vi "BuildCustomDashBoardData.vi"() -> ()   [LabVIEW 2013]
doc: "This VI builds data and sends it back to the dashboard PC program. By default it sends back the raw values for the first analog, digital, and solenoid module. Modify it to send back the data you want to view. Consider adding higher level data to the Dashboard Datatype.ctl and to this VI. Then update the Dashboard to display the data however you like.\n\nThis software is licensed. Open the labview\\readme\\WPI Robotics Library Open Source License.txt file for more information."
uses:
  typedefs/Dashboard/DashboardEnable.ctl
  <vilib>/Rock Robotics/SystemInterfaces/Typedef/FPGA_TypedefDigitalModule.ctl
  <vilib>/Rock Robotics/WPI/DriverStation/WPI_DriverStationDigitalData.ctl
  typedefs/fg_typedef.ctl
  typedefs/Dashboard/misc dash data.ctl
  typedefs/Dashboard/dashboard safety status data.ctl
  typedefs/Dashboard/drive safety.ctl
  typedefs/Dashboard/dash error type def.ctl
  <vilib>/Rock Robotics/SystemInterfaces/System/FPGA_SystemGet.vi
  <vilib>/Rock Robotics/WPI/Compressor/WPI_CompressorGetSetRefNum.vi
  <vilib>/NI_Real-Time Target Support.lvlib
  typedefs/State Machine/subStates.ctl
  typedefs/Dashboard/custom dash data.ctl
  typedefs/Dashboard/Dashboard Datatype.ctl
panel:
  out "Errors":errorcluster
  # "Generate Dashboard Data and Send it"
  # "Note: Test code calls some dashboard data, which is gotten there not here"
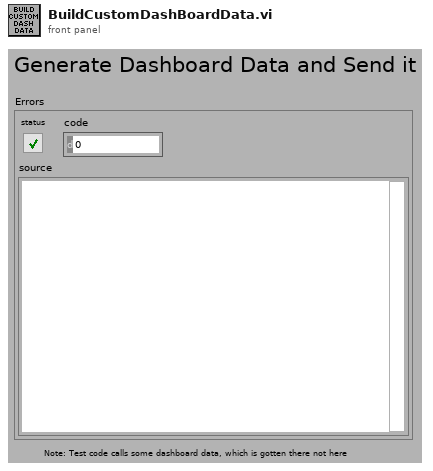
[diagram p1: front panel]
types:
  T1 = typedef "Dashboard Datatype.ctl" = cluster{cluster{"AnalogModule[0]":cluster{"Channel[0]":sgl, "Channel[1]":sgl, "Channel[2]":sgl, "Channel[3]":sgl, "Channel[4]":sgl, "Channel[5]":sgl, "Channel[6]":sgl, "Channel[7]":sgl}, "AnalogModule[1]":cluster{"Channel[0]":sgl, "Channel[1]":sgl, "Channel[2]":sgl, "Channel[3]":sgl, "Channel[4]":sgl, "Channel[5]":sgl, "Channel[6]":sgl, "Channel[7]":sgl}}, cluster{"DigitalModule[0]":T2, "DigitalModule[1]":T2}, "Solenoid":u8}
  T2 = typedef "WPI_DriverStationDigitalData.ctl" = cluster{"Relay Fwd":u8, "Relay Rev":u8, "GPIO":u16, "GPIO_OE":u16, "PWM":cluster{"PWM[0]":u8, "PWM[1]":u8, "PWM[2]":u8, "PWM[3]":u8, "PWM[4]":u8, "PWM[5]":u8, "PWM[6]":u8, "PWM[7]":u8, "PWM[8]":u8, "PWM[9]":u8}}
  T3 = typedef "custom dash data.ctl" = cluster{"Motors":cluster{"Pickup Motor":dbl, "Pickup Belt":dbl, "Pickup Distance ":dbl, "Pickup Rate":dbl, "Right Motor Rate":dbl, "Left Motor Rate":dbl, "Right Motor Distance":dbl, "Left Motor Distance":dbl}, "substates":cluster{"Latch":T4, "Pickup Arm":T4, "Belts":T4, "Shooter":T4, "Drive":T4}, "Safeties":cluster{"Arm Safety":bool, "Arm Limit":bool}, "Performance":cluster{"CPU Usage":dbl, "Vision mSPI":u32, "Main mSPI":u32}, "Vision Enabled?":bool, "Can Shoot Safely?":bool, "Timeout Error":cluster{"# of Timeouts":u32, "Time Out Error This Match":bool}, "Error FG Data":cluster{"Errors Present":bool, "Errors":string}, "Vision Data":cluster{"Hot Goal Present?":bool, "distance":dbl}}
  T4 = typedef "subStates.ctl" = enum16{"null", "wait", "driver control", "auto", "manual override", "hold position", "rotate", "pickup", "pass", "recover pass", "load", "goto shoot", "shoot high goal", "shoot low goal", "cancel arm", "cancel shooter", "end", "test"}
  T5 = typedef "fg_typedef.ctl" = enum16{"Get", "Set"}
  T6 = cluster{"# of Timeouts":u32, "Time Out Error This Match":bool}
  T7 = typedef "FPGA_TypedefDigitalModule.ctl" = enum16{"Digital Module 1", "Digital Module 2"}
  T8 = typedef "misc dash data.ctl" = cluster{"Total (%)":dbl, "Vision mSPI":u32, "Main mSPI":u32, "Vision":cluster{"Hot Goal Present?":bool, "distance":dbl}, "Enabled?":bool, "Arm Safety Data":T9, "Drive Safety Data":T10, "TeleOp Elapsed Seconds":dbl}
  T9 = typedef "dashboard safety status data.ctl" = cluster{"At Distance Limit":bool, "No Rate Read":bool, "Encoder Failure":bool, "Encoder Directional Issue":bool}
  T10 = typedef "drive safety.ctl" = cluster{"Left - Encoder Failure":bool, "Left - No Rate Read":bool, "Right - Encoder Failure":bool, "Right - No Rate Read":bool}
  T11 = typedef "dash error type def.ctl" = cluster{"Timeout Data":cluster{"# of Timeouts":u32, "Time Out Error This Match":bool}, "Can Shoot Safely?":bool}
  T12 = typedef "DashboardEnable.ctl" = cluster{"Analog Module 1":bool[], "Analog Module 2":bool[], "Digital Module 1":bool, "Digital Module 2":bool, "Solenoid Module":bool}
  T13 = cluster{"AnalogModule[0]":cluster{"Channel[0]":sgl, "Channel[1]":sgl, "Channel[2]":sgl, "Channel[3]":sgl, "Channel[4]":sgl, "Channel[5]":sgl, "Channel[6]":sgl, "Channel[7]":sgl}, "AnalogModule[1]":cluster{"Channel[0]":sgl, "Channel[1]":sgl, "Channel[2]":sgl, "Channel[3]":sgl, "Channel[4]":sgl, "Channel[5]":sgl, "Channel[6]":sgl, "Channel[7]":sgl}}
  T14 = cluster{"DigitalModule[0]":T2, "DigitalModule[1]":T2}
  T15 = typedef "vision data.ctl" = cluster{"x":dbl, "y":dbl, "area":dbl, "width":dbl, "height":dbl, "Hot Goal Present?":bool, "distance":dbl}
  T16 = cluster{"Channel[0]":sgl, "Channel[1]":sgl, "Channel[2]":sgl, "Channel[3]":sgl, "Channel[4]":sgl, "Channel[5]":sgl, "Channel[6]":sgl, "Channel[7]":sgl}[]
  T17 = cluster{"Channel[0]":sgl, "Channel[1]":sgl, "Channel[2]":sgl, "Channel[3]":sgl, "Channel[4]":sgl, "Channel[5]":sgl, "Channel[6]":sgl, "Channel[7]":sgl}
  T18 = cluster{"AnalogModule[0][0]":sgl, "AnalogModule[0][1]":sgl, "AnalogModule[0][2]":sgl, "AnalogModule[0][3]":sgl, "AnalogModule[0][4]":sgl, "AnalogModule[0][5]":sgl, "AnalogModule[0][6]":sgl, "AnalogModule[0][7]":sgl}
  T19 = cluster{"[0]":cluster{"Channel[0]":sgl, "Channel[1]":sgl, "Channel[2]":sgl, "Channel[3]":sgl, "Channel[4]":sgl, "Channel[5]":sgl, "Channel[6]":sgl, "Channel[7]":sgl}, "[1]":cluster{"Channel[0]":sgl, "Channel[1]":sgl, "Channel[2]":sgl, "Channel[3]":sgl, "Channel[4]":sgl, "Channel[5]":sgl, "Channel[6]":sgl, "Channel[7]":sgl}}
  T20 = typedef "FPGA_DIODevRef.ctl" = cluster{"DevStatus":errorcluster, "Module":T7}
  T21 = cluster{"[0]":u8, "[1]":u8, "[2]":u8, "[3]":u8, "[4]":u8, "[5]":u8, "[6]":u8, "[7]":u8, "[8]":u8, "[9]":u8}
  T22 = typedef "FPGA_SolenoidDevRef.ctl" = cluster{"DevStatus":errorcluster, "Module":T23}
  T23 = typedef "FPGA_TypedefSolenoidModule.ctl" = enum16{"Solenoid Module 1", "Solenoid Module 2"}
  T24 = cluster{"Pickup Motor":dbl, "Pickup Belt":dbl, "Pickup Distance ":dbl, "Pickup Rate":dbl, "Right Motor Rate":dbl, "Left Motor Rate":dbl, "Right Motor Distance":dbl, "Left Motor Distance":dbl}
  T25 = cluster{"CPU Usage":dbl, "Vision mSPI":u32, "Main mSPI":u32}
  T26 = cluster{"Hot Goal Present?":bool, "distance":dbl}
  T27 = typedef "WPI_EncoderDevRef.ctl" = cluster{"DevStatus":errorcluster, "EncoderIndex":T28, "CounterIndex":T29, "DistancePerCount":dbl, "Decoding Type":T30}
  T28 = typedef "FPGA_EncoderIdx.ctl" = enum8{"Enc 0", "Enc 1", "Enc 2", "Enc 3", "Invalid"}
  T29 = typedef "FPGA_CounterCtrSystemIndex.ctl" = enum8{"Ctr 0", "Ctr 1", "Ctr 2", "Ctr 3", "Ctr 4", "Ctr 5", "Ctr 6", "Ctr 7", "Invalid"}
  T30 = typedef "WPI_EncoderType.ctl" = enum16{"1x", "2x", "4x"}
  T31 = typedef "WPI_MotorControlDeviceRef.ctl" = cluster{"DeviceStatus":errorcluster, "Type":enum16{"PWM", "CAN"}, "PWM":cluster{"Digital Module":T7, "PWM Channel":T32, "DeadBand":T33}, "CAN":cluster{"Device Number":u8, "Control Mode":T34, "Semaphore":T35, "Max Vout":dbl}, "Invert":bool, "TransformRef":T36, "InvTransformRef":T36}
  T32 = typedef "FPGA_DIOPWMChannel.ctl" = enum8{"PWM 1", "PWM 2", "PWM 3", "PWM 4", "PWM 5", "PWM 6", "PWM 7", "PWM 8", "PWM 9", "PWM 10", "Invalid"}
  T33 = typedef "WPI_PWMDeadband.ctl" = cluster{"Name":string, "maxPositivePwm":i32, "minPositivePwm":i32, "centerPwm":i32, "maxNegativePwm":i32, "minNegativePwm":i32, "angularRange":u16}
  T34 = typedef "WPI_CANJaguar_ControlMode.ctl" = enum8{"Percent VBus", "Current", "Speed", "Position", "Voltage"}
  T35 = typedef "Semaphore RefNum" = refnum<k1>
  T36 = typedef "WPI_PWMTransform_ConPane.ctl" = refnum<vi>
  T37 = typedef "NI_Real-Time Target Support.lvlib/RT CPU Load.ctl" = cluster{"Total (%)":dbl, "Time Critical (%)":dbl, "Timed Structures (%)":dbl, "High (%)":dbl, "Above Normal (%)":dbl, "Normal (%)":dbl, "Background (%)":dbl, "Idle (%)":dbl, "ISR (%)":dbl}
  T38 = cluster{"Vision mSPI":u32, "Main mSPI":u32, "Dash mSPI":u32}
  T39 = typedef "WPI_CompressorDevRef.ctl" = cluster{"DevStatus":errorcluster, "DigitalInputDevRef":T40, "RelayDevRef":T42}
  T40 = typedef "WPI_DigitalInputDevRef.ctl" = cluster{"DevStatus":errorcluster, "DIO Channel":T41, "Digital Module":T7}
  T41 = typedef "FPGA_DIOChannel.ctl" = enum8{"DIO 1", "DIO 2", "DIO 3", "DIO 4", "DIO 5", "DIO 6", "DIO 7", "DIO 8", "DIO 9", "DIO 10", "DIO 11", "DIO 12", "DIO 13", "DIO 14", "Invalid"}
  T42 = typedef "WPI_RelayDevRef.ctl" = cluster{"DevStatus":errorcluster, "Relay Channel":T43, "Digital Module":T7, "Relay Direction":T44}
  T43 = typedef "FPGA_DIORelayChannel.ctl" = enum8{"Relay 1", "Relay 2", "Relay 3", "Relay 4", "Relay 5", "Relay 6", "Relay 7", "Relay 8", "Invalid"}
  T44 = typedef "WPI_RelayDirection.ctl" = enum16{"Both directions", "Forward only", "Reverse only"}
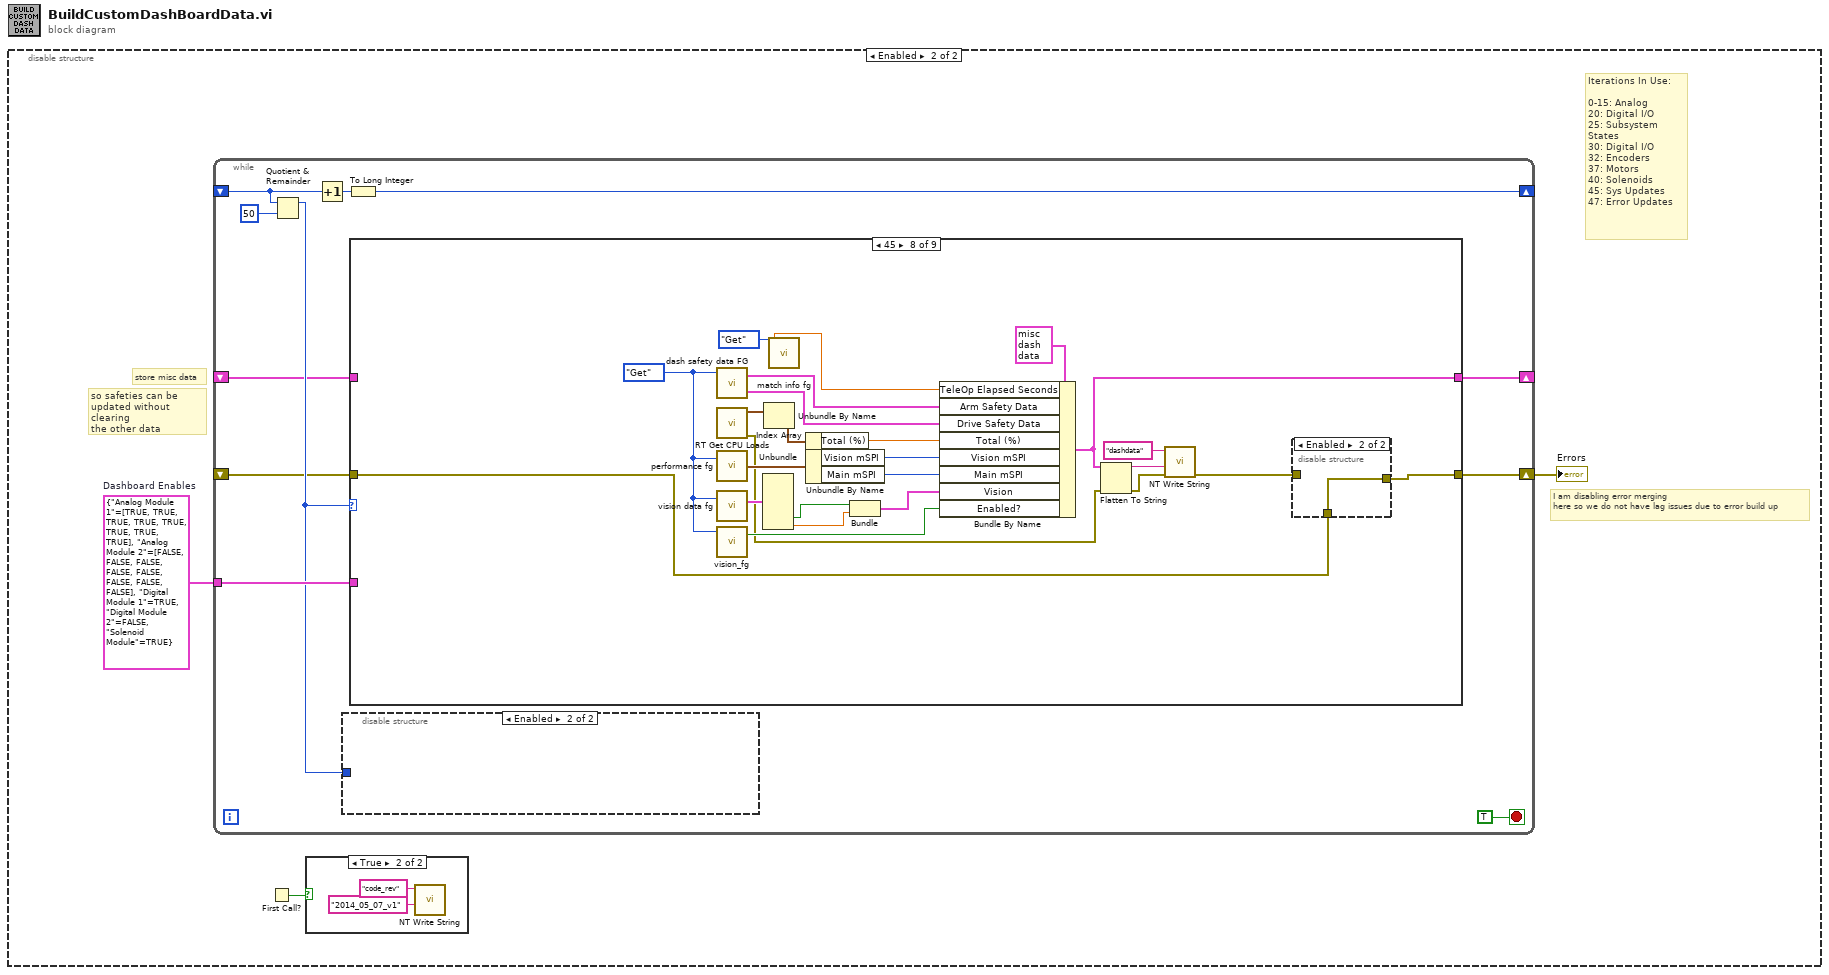
[diagram p0: block diagram]
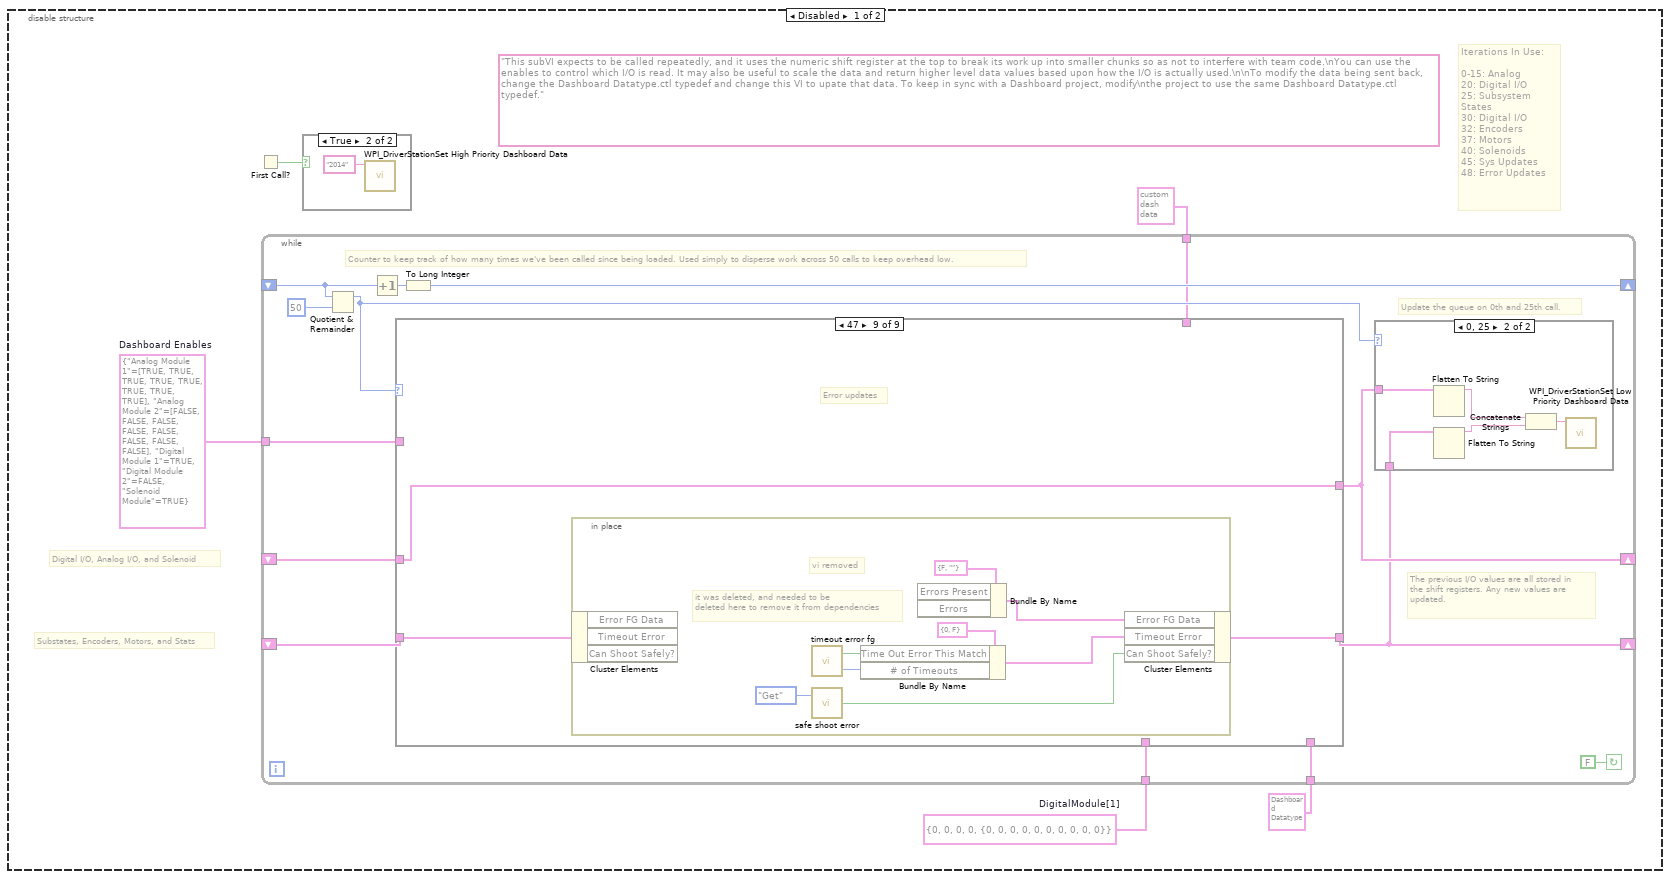
[diagram p2: hidden frame]
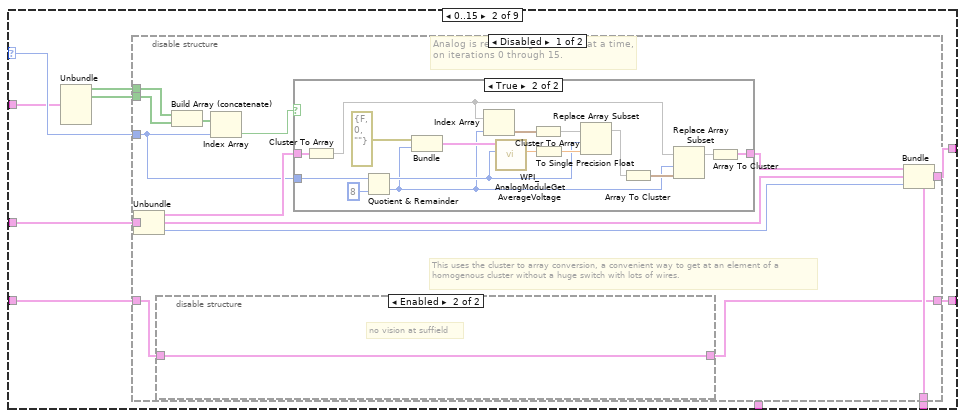
[diagram p6: hidden frame]
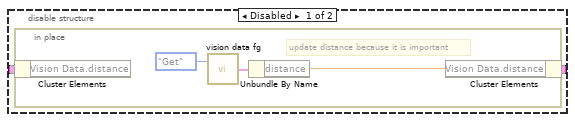
[diagram p8: hidden frame]
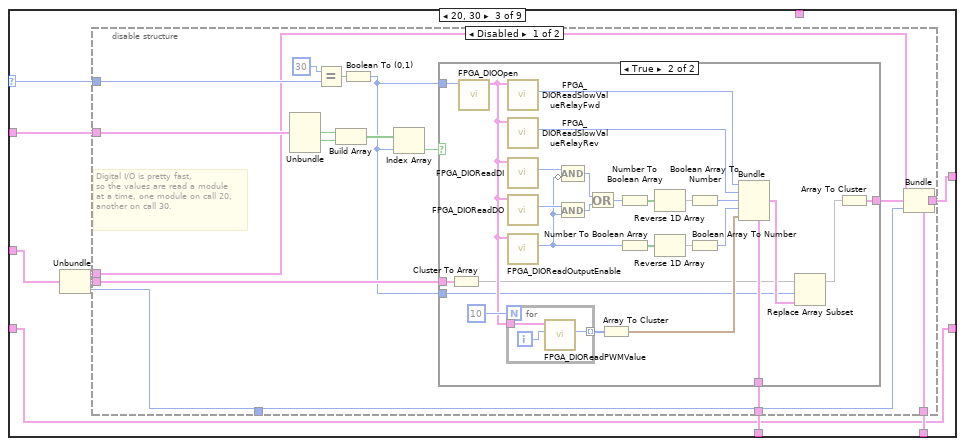
[diagram p10: hidden frame]
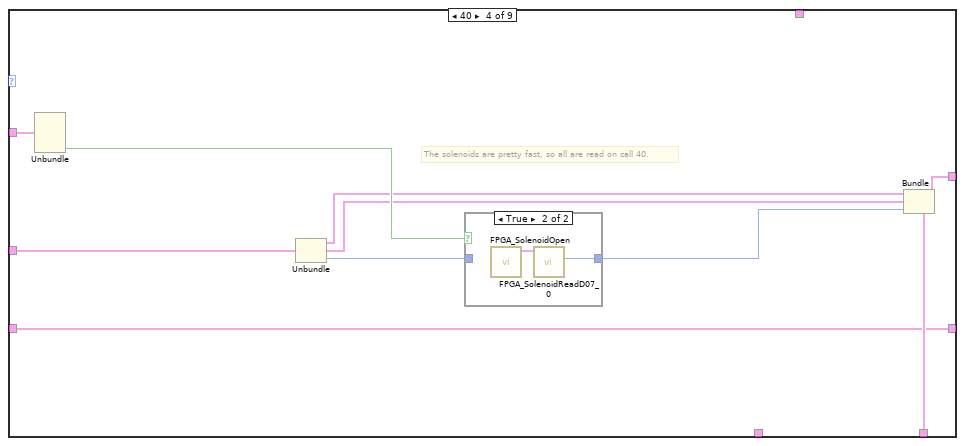
[diagram p13: hidden frame]
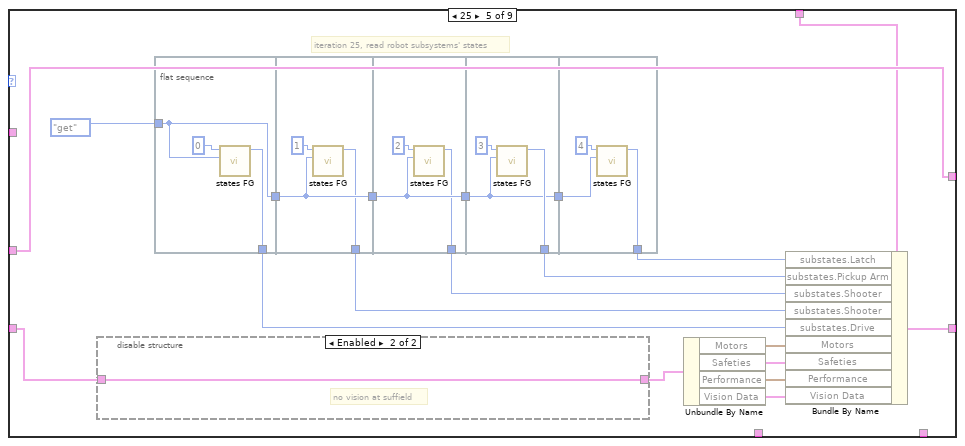
[diagram p15: hidden frame]
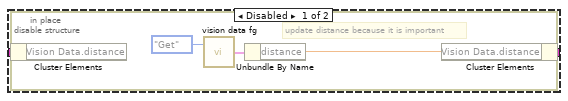
[diagram p16: hidden frame]
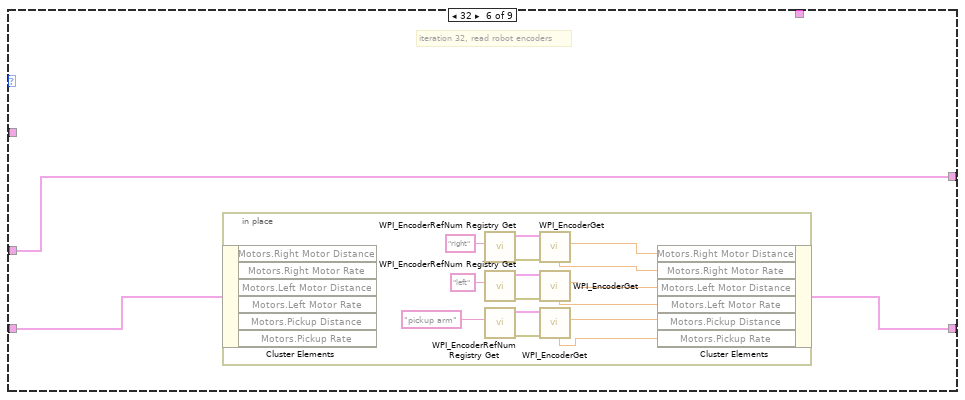
[diagram p17: hidden frame]
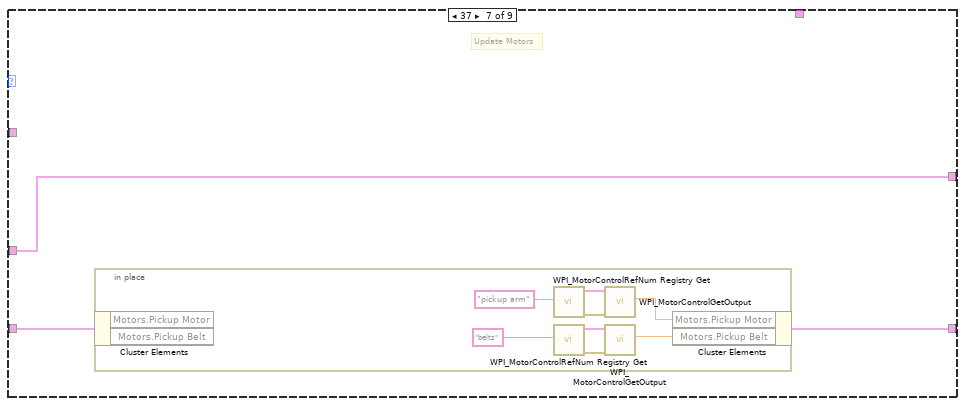
[diagram p18: hidden frame]
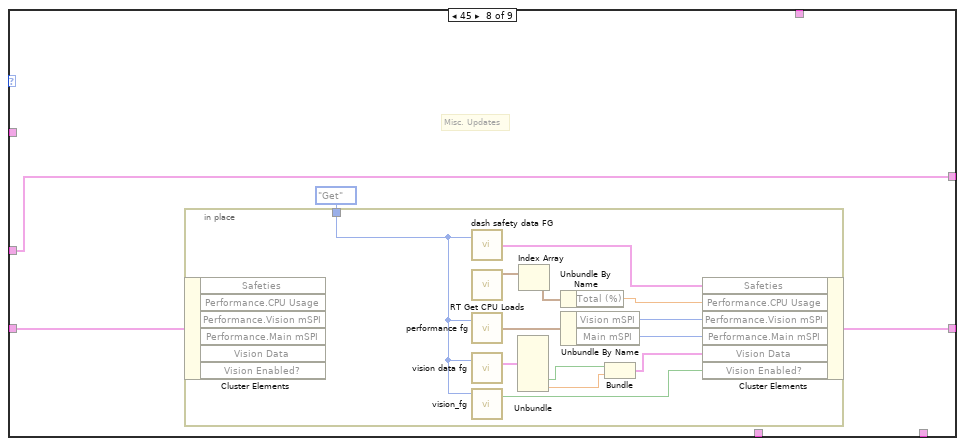
[diagram p19: hidden frame]
diagram:
  n1 = disable-structure shown="Enabled" {
    frame Disabled {
      w1 = T12 {"Analog Module 1"=[TRUE, TRUE, TRUE, TRUE, TRUE, TRUE, TRUE, TRUE], "Analog Module 2"=[FALSE, FALSE, FALSE, FALSE, FALSE, FALSE, FALSE, FALSE], "Digital Module 1"=TRUE, "Digital Module 2"=FALSE, "Solenoid Module"=TRUE}  # Dashboard Enables
      w2 = T2 {"Relay Fwd"=0, "Relay Rev"=0, "GPIO"=0, "GPIO_OE"=0, "PWM"={"PWM[0]"=0, "PWM[1]"=0, "PWM[2]"=0, "PWM[3]"=0, "PWM[4]"=0, "PWM[5]"=0, "PWM[6]"=0, "PWM[7]"=0, "PWM[8]"=0, "PWM[9]"=0}}  # DigitalModule[1]
      (unwired) "This subVI expects to be called repeatedly, and it uses the numeric shift register at the top to break its work up into smaller chunks so as not to interfere with team code.\nYou can use the enables to control which I/O is read. It may also be useful to scale the data and return higher level data values based upon how the I/O is actually used.\n\nTo modify the data being sent back, change the Dashboard Datatype.ctl typedef and change this VI to upate that data. To keep in sync with a Dashboard project, modify\nthe project to use the same Dashboard Datatype.ctl typedef."
      # "Iterations In Use:\n\n0-15: Analog\n20: Digital I/O \n25: Subsystem States\n30: Digital I/O\n32: Encoders\n37: Motors\n40: Solenoids\n45: Sys Updates\n48: Error Updates"
      # "Substates, Encoders, Motors, and Stats"
      # "Digital I/O, Analog I/O, and Solenoid"
      n2 = First Call?() -> (First Call?: T/F=w3:bool)
      n3 = while {
        shift-right: [w13] -> _
        shift-left: _ -> [w15]
        shift-right: [w10] -> _
        shift-left: _ -> [w18]
        tunnel: w2 -> [w17]
        tunnel: T1 {{"AnalogModule[0]"={"Channel[0]"=0.0, "Channel[1]"=0.0, "Channel[2]"=0.0, "Channel[3]"=0.0, "Channel[4]"=0.0, "Channel[5]"=0.0, "Channel[6]"=0.0, "Channel[7]"=0.0}, "AnalogModule[1]"={"Channel[0]"=0.0, "Channel[1]"=0.0, "Channel[2]"=0.0, "Channel[3]"=0.0, "Channel[4]"=0.0, "Channel[5]"=0.0, "Channel[6]"=0.0, "Channel[7]"=0.0}}, {"DigitalModule[0]"={"Relay Fwd"=0, "Relay Rev"=0, "GPIO"=0, "GPIO_OE"=0, "PWM"={"PWM[0]"=0, "PWM[1]"=0, "PWM[2]"=0, "PWM[3]"=0, "PWM[4]"=0, "PWM[5]"=0, "PWM[6]"=0, "PWM[7]"=0, "PWM[8]"=0, "PWM[9]"=0}}, "DigitalModule[1]"={"Relay Fwd"=0, "Relay Rev"=0, "GPIO"=0, "GPIO_OE"=0, "PWM"={"PWM[0]"=0, "PWM[1]"=0, "PWM[2]"=0, "PWM[3]"=0, "PWM[4]"=0, "PWM[5]"=0, "PWM[6]"=0, "PWM[7]"=0, "PWM[8]"=0, "PWM[9]"=0}}}, "Solenoid"=0} ("Dashboard Data") -> [w12]
        tunnel: w1 -> [w11]
        shift-right: [w7] -> _
        shift-left: _ -> [w8]
        tunnel: T3 {"Motors"={"Pickup Motor"=0.0, "Pickup Belt"=0.0, "Pickup Distance "=0.0, "Pickup Rate"=0.0, "Right Motor Rate"=0.0, "Left Motor Rate"=0.0, "Right Motor Distance"=0.0, "Left Motor Distance"=0.0}, "substates"={"Latch"=enum."null", "Pickup Arm"=enum."null", "Belts"=enum."null", "Shooter"=enum."null", "Drive"=enum."null"}, "Safeties"={"Arm Safety"=FALSE, "Arm Limit"=FALSE}, "Performance"={"CPU Usage"=0.0, "Vision mSPI"=0, "Main mSPI"=0}, "Vision Enabled?"=FALSE, "Can Shoot Safely?"=FALSE, "Timeout Error"={"# of Timeouts"=0, "Time Out Error This Match"=FALSE}, "Error FG Data"={"Errors Present"=FALSE, "Errors"=""}, "Vision Data"={"Hot Goal Present?"=FALSE, "distance"=0.0}} ("Custom Dash Data") -> [w9]
        stop <- FALSE continue-if-true
        # "Counter to keep track of how many times we've been called since being loaded. Used simply to disperse work across 50 calls to keep overhead low."
        # "Update the queue on 0th and 25th call."
        # "The previous I/O values are all stored in\nthe shift registers. Any new values are\nupdated."
        n4 = Quotient & Remainder(x=w15, y=50) -> (x-y*floor(x/y)=w14:i32)  [unwired: 1 out]
        n5 = Increment(x=w15) -> (x+1=w20:i32)
        n6 = case shown="47" w14 {
          selector: w14 -> [_ w35 w82 _ _ _ _ _ _]
          tunnel: [w27 w31 w77 w136 w151 w184 w203 w214 w230] -> w10
          tunnel: w18 -> [w27 w30 w79 w138 w151 w184 w203 w214 w230]
          tunnel: w17 -> [_ _ w83 _ _ _ _ _ _]
          tunnel: w12 -> [_ w36 w78 w135 _ _ _ _ _]
          tunnel: w11 -> [_ w34 w81 w139 _ _ _ _ _]
          tunnel: w9 -> [_ _ _ _ w149 _ _ _ _]
          tunnel: [w26 w28 w76 w132 w150 w185 w202 w215 w231] -> w7
          tunnel: w8 -> [w26 w29 w76 w132 w145 w183 w201 w213 w229]
          frame Default {
            # "Don't update any I/O"
          }
          frame 0..15 {
            n7 = Unbundle(w34) -> ("Analog Module 1"=w33:bool[], "Analog Module 2"=w32:bool[])  [unwired: 3 out]
            n8 = disable-structure shown="Disabled" {
              disable-tunnel: w36 -> [w47 _]
              disable-tunnel: w35 -> [w45 _]
              disable-tunnel: w33 -> [w44 _]
              disable-tunnel: w32 -> [w43 _]
              disable-tunnel: [w42 _] -> w31
              disable-tunnel: w30 -> [w41 _]
              disable-tunnel: w29 -> [w38 _]
              disable-tunnel: [w37 _] -> w28
              frame Disabled {
                # "This uses the cluster to array conversion, a convenient way to get at an element of a\nhomogenous cluster without a huge switch with lots of wires."
                # "Analog is read a single channel at a time,\non iterations 0 through 15."
                n9 = Unbundle(w41) -> (w46:T13, w40:T14, "Solenoid"=w39:u8)
                n10 = disable-structure shown="Enabled" {
                  disable-tunnel: w38 -> [w69 w73]
                  disable-tunnel: [w68 w73] -> w37
                  frame Disabled {
                    n11 = in-place {
                      # "update distance because it is important"
                      n12 = in-place-cluster #1(w69) -> ()  [unwired: 1 out]
                      n13 = call "vision data fg.vi"("Menu"=fg_typedef."Get") -> ("Output"=w71:T15)  [unwired: 1 in]
                      n14 = Unbundle By Name(w71) -> ("distance"=w70:dbl)
                      n15 = in-place-cluster #1("Vision Data.distance"=w70) -> (w68:T3)
                    }
                  }
                  frame Enabled {
                    # "no vision at suffield"
                  }
                }
                n16 = Build Array (concatenate)(w44, w43) -> (w49:bool[])
                n17 = Index Array(array=w49, index=w45) -> (element=w50:bool)
                n18 = case shown="True" w50 {
                  tunnel: w45 -> [_ w58]
                  tunnel: [w51 w55] -> w48
                  tunnel: w46 -> [w51 w54]
                  frame False {
                  }
                  frame True {
                    n19 = Cluster To Array(cluster=w54) -> (array=w53:T16)
                    n20 = Quotient & Remainder(x=w58, y=8) -> (x-y*floor(x/y)=w57:i32, floor(x/y)=w52:i32)
                    n21 = Bundle("DevStatus"=errorcluster {"status"=FALSE, "code"=0, "source"=""}, w52) -> (w66:cluster{"DevStatus":errorcluster, i32})  [unwired: 1 out]
                    n22 = Index Array(array=w53, index=w52) -> (element=w60:T17)
                    n23 = call <vilib>:"WPI_AnalogModuleGetAverageVoltage.vi"("Channel"=w57, "AnalogModuleDevStatus"=w66) -> ("Average Voltage"=w63:dbl)  [unwired: 1 in, 8 out]
                    n24 = Cluster To Array(cluster=w60) -> (array=w59:sgl[])
                    n25 = To Single Precision Float(number=w63) -> (single precision float=w62:sgl)
                    n26 = Replace Array Subset(array=w59, new element=w62, index=w57) -> (w61:sgl[])
                    n27 = Array To Cluster(array=w61) -> (cluster=w65:T18)
                    n28 = Replace Array Subset(array=w53, new element=w65, index=w52) -> (w56:T16)
                    n29 = Array To Cluster(array=w56) -> (cluster=w55:T19)
                  }
                }
                n30 = Bundle(cluster=w47, w48, w40, "Solenoid"=w39) -> (w42:T1)
              }
              frame Enabled {
              }
            }
          }
          frame 20, 30 {
            n31 = Unbundle(w79) -> (w75:T13, w80:T14, "Solenoid"=w74:u8)
            n32 = disable-structure shown="Disabled" {
              disable-tunnel: w83 -> [w99 _]
              disable-tunnel: w82 -> [w95 _]
              disable-tunnel: w81 -> [w93 _]
              disable-tunnel: w80 -> [w90 _]
              disable-tunnel: w78 -> [w88 _]
              disable-tunnel: [w87 _] -> w77
              disable-tunnel: w75 -> [w85 _]
              disable-tunnel: w74 -> [w84 _]
              frame Disabled {
                # "Digital I/O is pretty fast,\nso the values are read a module\nat a time, one module on call 20,\nanother on call 30."
                n33 = Unbundle(w93) -> ("Digital Module 1"=w92:bool, "Digital Module 2"=w91:bool)  [unwired: 3 out]
                n34 = Equal?(x=30, y=w95) -> (x = y?=w97:bool)
                n35 = Build Array(w92, w91) -> (w94:bool[])
                n36 = Boolean To (0,1)(Boolean=w97) -> (0, 1=w86:i16)
                n37 = Index Array(array=w94, index=w86) -> (element=w96:bool)
                n38 = case shown="True" w96 {
                  tunnel: w99 -> [_ w108]
                  tunnel: [w100 w101] -> w89
                  tunnel: w86 -> [_ w106]
                  tunnel: w86 -> [_ w105]
                  tunnel: w90 -> [w100 w104]
                  frame False {
                  }
                  frame True {
                    n39 = Cluster To Array(cluster=w104) -> (array=w103:T2[])
                    n40 = call <vilib>:"FPGA_DIOOpen.vi"("Module (Module 1)"=w106) -> ("DIODeviceRef"=w124:T20)  [unwired: 1 in, 9 out]
                    n41 = for {
                      N: 10 -> [_]
                      tunnel: w124 -> [w129]
                      tunnel: [w127] -> w125 mode=indexing
                      i -> [w128]
                      n42 = call <vilib>:"FPGA_DIOReadPWMValue.vi"("PWMChannel"=w128, "DIODeviceRef In"=w129) -> ("PWMValue"=w127:u8)  [unwired: 1 in, 8 out]
                    }
                    n43 = call <vilib>:"FPGA_DIOReadSlowValueRelayFwd.vi"("DIODeviceRef In"=w124) -> ("Relay Forward"=w117:u8)  [unwired: 1 in, 9 out]
                    n44 = call <vilib>:"FPGA_DIOReadSlowValueRelayRev.vi"("DIODeviceRef In"=w124) -> ("Relay Reverse"=w118:u8)  [unwired: 1 in, 9 out]
                    n45 = call <vilib>:"FPGA_DIOReadDI.vi"("DIODeviceRef In"=w124) -> ("DI"=w122:u16)  [unwired: 1 in, 9 out]
                    n46 = call <vilib>:"FPGA_DIOReadDO.vi"("DIODeviceRef In"=w124) -> ("DO"=w121:u16)  [unwired: 1 in, 9 out]
                    n47 = call <vilib>:"FPGA_DIOReadOutputEnable.vi"("DIODeviceRef In"=w124) -> ("OutputEnable"=w112:u16)  [unwired: 1 in, 9 out]
                    n48 = And(x=w121, y=w112) -> (x .and. y?=w120:u16)
                    n49 = Compound Arithmetic op=AND(w122, invert w112) -> (w119:u16)
                    n50 = Or(x=w119, y=w120) -> (x .or. y?=w110:u16)
                    n51 = Array To Cluster(array=w125) -> (cluster=w123:T21)
                    n52 = Number To Boolean Array(number=w110) -> (Boolean array=w115:bool[])
                    n53 = Number To Boolean Array(number=w112) -> (Boolean array=w114:bool[])
                    n54 = Reverse 1D Array(array=w115) -> (reversed array=w116:bool[])
                    n55 = Reverse 1D Array(array=w114) -> (reversed array=w113:bool[])
                    n56 = Boolean Array To Number(Boolean array=w116) -> (number=w109:u32)
                    n57 = Boolean Array To Number(Boolean array=w113) -> (number=w111:u32)
                    n58 = Bundle(cluster=w108, "Relay Fwd"=w117, "Relay Rev"=w118, "GPIO"=w109, "GPIO_OE"=w111, "PWM"=w123) -> (w107:T2)
                    n59 = Replace Array Subset(array=w103, new element=w107, index=w105) -> (w102:T2[])
                    n60 = Array To Cluster(array=w102) -> (cluster=w101:cluster{"[0]":T2, "[1]":T2})
                  }
                }
                n61 = Bundle(cluster=w88, w85, w89, "Solenoid"=w84) -> (w87:T1)
              }
              frame Enabled {
              }
            }
          }
          frame 40 {
            # "The solenoids are pretty fast, so all are read on call 40."
            n62 = Unbundle(w139) -> ("Solenoid Module"=w133:bool)  [unwired: 4 out]
            n63 = Unbundle(w138) -> (w131:T13, w130:T14, "Solenoid"=w137:u8)
            n64 = case shown="True" w133 {
              tunnel: [w140 w141] -> w134
              tunnel: w137 -> [w140 _]
              frame False {
              }
              frame True {
                n65 = call <vilib>:"FPGA_SolenoidOpen.vi"() -> ("SolenoidDevRef"=w142:T22)  [unwired: 2 in, 9 out]
                n66 = call <vilib>:"FPGA_SolenoidReadD07_0.vi"("SolenoidDevRef"=w142) -> ("DO7:0"=w141:u8)  [unwired: 1 in, 9 out]
              }
            }
            n67 = Bundle(cluster=w135, w131, w130, "Solenoid"=w134) -> (w136:T1)
          }
          frame 25 {
            # "iteration 25, read robot subsystems' states"
            n68 = disable-structure shown="Enabled" {
              disable-tunnel: w145 -> [w163 w167]
              disable-tunnel: [w162 w167] -> w144
              frame Disabled {
                n69 = in-place {
                  # "update distance because it is important"
                  n70 = in-place-cluster #2(w163) -> ()  [unwired: 1 out]
                  n71 = call "vision data fg.vi"("Menu"=fg_typedef."Get") -> ("Output"=w165:T15)  [unwired: 1 in]
                  n72 = Unbundle By Name(w165) -> ("distance"=w164:dbl)
                  n73 = in-place-cluster #2("Vision Data.distance"=w164) -> (w162:T3)
                }
              }
              frame Enabled {
                # "no vision at suffield"
              }
            }
            n74 = flat-sequence {
              tunnel: enum16{"set", "get"}."get" ("menu (get)") -> [w170]
              tunnel: [w170] -> w158
              tunnel: [w168] -> w152
              tunnel: [w173] -> w159
              tunnel: w158 -> [w173]
              tunnel: [w171] -> w153
              tunnel: [w176] -> w160
              tunnel: w159 -> [w176]
              tunnel: [w174] -> w154
              tunnel: w160 -> [w177]
              tunnel: [w178] -> w155
              tunnel: [w177] -> w157
              tunnel: w157 -> [w181]
              tunnel: [w180] -> w156
              frame #0 {
                n75 = call "states FG.vi"("menu (get)"=w170, "Loop ID"=0) -> ("subState out"=w168:T4)  [unwired: 6 in, 3 out]
              }
              frame #1 {
                n76 = call "states FG.vi"("menu (get)"=w173, "Loop ID"=1) -> ("subState out"=w171:T4)  [unwired: 6 in, 3 out]
              }
              frame #2 {
                n77 = call "states FG.vi"("menu (get)"=w176, "Loop ID"=2) -> ("subState out"=w174:T4)  [unwired: 6 in, 3 out]
              }
              frame #3 {
                n78 = call "states FG.vi"("menu (get)"=w177, "Loop ID"=3) -> ("subState out"=w178:T4)  [unwired: 6 in, 3 out]
              }
              frame #4 {
                n79 = call "states FG.vi"("menu (get)"=w181, "Loop ID"=4) -> ("subState out"=w180:T4)  [unwired: 6 in, 3 out]
              }
            }
            n80 = Unbundle By Name(w144) -> ("Motors"=w143:T24, "Safeties"=w148:cluster{"Arm Safety":bool, "Arm Limit":bool}, "Performance"=w147:T25, "Vision Data"=w146:T26)
            n81 = Bundle By Name(cluster=w149, "substates.Latch"=w156, "substates.Pickup Arm"=w155, "substates.Shooter"=w154, "substates.Shooter"=w153, "substates.Drive"=w152, "Motors"=w143, "Safeties"=w148, "Performance"=w147, "Vision Data"=w146) -> (w150:T3)
          }
          frame 32 {
            # "iteration 32, read robot encoders"
            n82 = in-place {
              n83 = in-place-cluster #3(w183) -> ()  [unwired: 6 out]
              n84 = call <vilib>:"WPI_EncoderRefNum Registry Get.vi"("refnum name"="right") -> ("error out"=w192:errorcluster, "EncoderDevRef"=w193:T27)  [unwired: 9 in]
              n85 = call <vilib>:"WPI_EncoderRefNum Registry Get.vi"("refnum name"="left") -> ("error out"=w195:errorcluster, "EncoderDevRef"=w194:T27)  [unwired: 9 in]
              n86 = call <vilib>:"WPI_EncoderRefNum Registry Get.vi"("refnum name"="pickup arm") -> ("error out"=w199:errorcluster, "EncoderDevRef"=w200:T27)  [unwired: 9 in]
              n87 = call <vilib>:"WPI_EncoderGet.vi"("error in (no error)"=w192, "EncoderDevRef"=w193) -> ("Distance"=w187:dbl, "Rate"=w186:dbl)  [unwired: 4 in, 4 out]
              n88 = call <vilib>:"WPI_EncoderGet.vi"("error in (no error)"=w195, "EncoderDevRef"=w194) -> ("Distance"=w188:dbl, "Rate"=w189:dbl)  [unwired: 4 in, 4 out]
              n89 = call <vilib>:"WPI_EncoderGet.vi"("error in (no error)"=w199, "EncoderDevRef"=w200) -> ("Distance"=w197:dbl, "Rate"=w196:dbl)  [unwired: 4 in, 4 out]
              n90 = in-place-cluster #3("Motors.Right Motor Distance"=w187, "Motors.Right Motor Rate"=w186, "Motors.Left Motor Distance"=w188, "Motors.Left Motor Rate"=w189, "Motors.Pickup Distance"=w197, "Motors.Pickup Rate"=w196) -> (w185:T3)
            }
          }
          frame 37 {
            # "Update Motors"
            n91 = in-place {
              n92 = in-place-cluster #4(w201) -> ()  [unwired: 2 out]
              n93 = call <vilib>:"WPI_MotorControlRefNum Registry Get.vi"("refnum name"="pickup arm") -> ("error out"=w204:errorcluster, "MotorControlDevRef"=w208:T31)  [unwired: 9 in]
              n94 = call <vilib>:"WPI_MotorControlRefNum Registry Get.vi"("refnum name"="belts") -> ("error out"=w205:errorcluster, "MotorControlDevRef"=w211:T31)  [unwired: 9 in]
              n95 = call <vilib>:"WPI_MotorControlGetOutput.vi"("error in (no error)"=w204, "MotorControlDevRef"=w208) -> ("Output"=w207:dbl)  [unwired: 7 in, 2 out]
              n96 = call <vilib>:"WPI_MotorControlGetOutput.vi"("error in (no error)"=w205, "MotorControlDevRef"=w211) -> ("Output"=w206:dbl)  [unwired: 7 in, 2 out]
              n97 = in-place-cluster #4("Motors.Pickup Motor"=w207, "Motors.Pickup Belt"=w206) -> (w202:T3)
            }
          }
          frame 45 {
            # "Misc. Updates"
            n98 = in-place {
              in-place-border: fg_typedef."Get" ("Menu (Get)") -> [w220]
              n99 = in-place-cluster #5(w213) -> ()  [unwired: 6 out]
              n100 = call "dash safety data FG.vi"("Menu"=w220) -> ("Safety Data Out"=w222:T9)  [unwired: 1 in]
              n101 = call <vilib>:"RT Get CPU Loads.vi"() -> ("CPU loads"=w227:T37[])  [unwired: 10 in, 1 out]
              n102 = call "performance fg.vi"("Menu"=w220) -> ("Output"=w223:T38)  [unwired: 1 in]
              n103 = call "vision data fg.vi"("Menu"=w220) -> ("Output"=w219:T15)  [unwired: 1 in]
              n104 = call "vision_fg.vi"("Menu"=w220) -> ("Enabled?"=w221:bool)  [unwired: 2 in, 1 out]
              n105 = Unbundle(w219) -> ("Hot Goal Present?"=w218:bool, "distance"=w217:dbl)  [unwired: 5 out]
              n106 = Index Array(array=w227) -> (element=w228:T37)  [unwired: 1 in]
              n107 = Unbundle By Name(w228) -> ("Total (%)"=w226:dbl)
              n108 = Unbundle By Name(w223) -> ("Vision mSPI"=w225:u32, "Main mSPI"=w224:u32)
              n109 = Bundle("Hot Goal Present?"=w218, "distance"=w217) -> (w216:T26)  [unwired: 1 in]
              n110 = in-place-cluster #5("Safeties"=w222, "Performance.CPU Usage"=w226, "Performance.Vision mSPI"=w225, "Performance.Main mSPI"=w224, "Vision Data"=w216, "Vision Enabled?"=w221) -> (w215:T3)
            }
          }
          frame 47 {
            # "Error updates"
            n111 = in-place {
              # "it was deleted, and needed to be\ndeleted here to remove it from dependencies"
              # "vi removed"
              n112 = in-place-cluster #6(w229) -> ()  [unwired: 3 out]
              n113 = call "timeout error fg.vi"() -> ("# of Timeouts"=w238:u32, "Time Out Error This Match"=w237:bool)  [unwired: 2 in]
              n114 = call "safe shoot error.vi"("Menu"=fg_typedef."Get") -> ("Can Shoot Safely?"=w234:bool)  [unwired: 1 in]
              n115 = Bundle By Name(cluster=T6 {"# of Timeouts"=0, "Time Out Error This Match"=FALSE}, "Time Out Error This Match"=w237, "# of Timeouts"=w238) -> (w236:T6)
              n116 = Bundle By Name(cluster=cluster{"Errors Present":bool, "Errors":string} {"Errors Present"=FALSE, "Errors"=""}) -> (w232:cluster{"Errors Present":bool, "Errors":string})  [unwired: 2 in]
              n117 = in-place-cluster #6("Error FG Data"=w232, "Timeout Error"=w236, "Can Shoot Safely?"=w234) -> (w231:T3)
            }
          }
        }
        n118 = To Long Integer(number=w20) -> (32bit integer=w13:i32)
        n119 = case shown="0, 25" w14 {
          tunnel: w10 -> [_ w25]
          tunnel: w7 -> [_ w23]
          frame Default {
          }
          frame 0, 25 {
            n120 = Flatten To String(anything=w25) -> (data string=w24:string)  [unwired: 1 in, 4 out]
            n121 = Flatten To String(anything=w23) -> (data string=w21:string)  [unwired: 1 in, 4 out]
            n122 = Concatenate Strings(w24, w21) -> (w22:string)
            n123 = call <vilib>:"WPI_DriverStationSet Low Priority Dashboard Data.vi"("User Data"=w22) -> ()  [unwired: 1 in, 10 out]
          }
        }
      }
      n124 = case shown="True" w3 {
        frame False {
        }
        frame True {
          n125 = call <vilib>:"WPI_DriverStationSet High Priority Dashboard Data.vi"("User Data"="2014") -> ()  [unwired: 10 in, 1 out]
        }
      }
    }
    frame Enabled {
      w242 = T12 {"Analog Module 1"=[TRUE, TRUE, TRUE, TRUE, TRUE, TRUE, TRUE, TRUE], "Analog Module 2"=[FALSE, FALSE, FALSE, FALSE, FALSE, FALSE, FALSE, FALSE], "Digital Module 1"=TRUE, "Digital Module 2"=FALSE, "Solenoid Module"=TRUE}  # Dashboard Enables
      # "I am disabling error merging\nhere so we do not have lag issues due to error build up"
      # "so safeties can be\nupdated without clearing\nthe other data"
      # "store misc data"
      # "Iterations In Use:\n\n0-15: Analog\n20: Digital I/O \n25: Subsystem States\n30: Digital I/O\n32: Encoders\n37: Motors\n40: Solenoids\n45: Sys Updates\n47: Error Updates"
      n126 = while {
        shift-right: [w252] -> _
        shift-left: _ -> [w253]
        tunnel: w242 -> [w250]
        shift-right: [w248] -> w241
        shift-left: _ -> [w247]
        shift-right: [w246] -> _
        shift-left: _ -> [w245]
        stop <- TRUE stop-if-true
        n127 = Quotient & Remainder(x=w253, y=50) -> (x-y*floor(x/y)=w249:i32)  [unwired: 1 out]
        n128 = Increment(x=w253) -> (x+1=w254:i32)
        n129 = disable-structure shown="Enabled" {
          disable-tunnel: w249 -> [w256 _]
          frame Disabled {
            n130 = case shown="10, 20, 30, 40, 50" w256 {
              frame 0, Default {
              }
              frame 10, 20, 30, 40, 50 {
                n131 = call "vision data fg.vi"("Menu"=fg_typedef."Get") -> ("Output"=w259:T15)  [unwired: 1 in]
                n132 = Unbundle By Name(w259) -> ("distance"=w258:dbl)
                n133 = call <vilib>:"NT Write Number.vi"("Numeric"=w258, "Name"="distance") -> ()  [unwired: 9 in, 1 out]
              }
            }
          }
          frame Enabled {
          }
        }
        n134 = To Long Integer(number=w254) -> (32bit integer=w252:i32)
        n135 = case shown="45" w249 {
          selector: w249 -> [_ w267 _ w339 _ _ _ _ _]
          tunnel: w250 -> [_ w268 _ w338 _ _ w447 _ _]
          tunnel: [w262 w266 w304 w329 w389 w416 w440 w467 w493] -> w248
          tunnel: w247 -> [w262 w265 w303 w330 w388 w415 w436 w466 w491]
          tunnel: [w261 w263 w302 w328 w387 w412 w435 w465 w490] -> w246
          tunnel: w245 -> [w261 w264 w302 w328 w387 w412 w435 _ w490]
          frame Default {
          }
          frame 0..15 {
            n136 = disable-structure shown="Disabled" {
              disable-tunnel: w268 -> [w275 _]
              disable-tunnel: w267 -> [w272 _]
              disable-tunnel: [w270 w299] -> w266
              disable-tunnel: w265 -> [w269 w299]
              disable-tunnel: w264 -> [_ w295]
              disable-tunnel: [_ w294] -> w263
              frame Enabled {
                # "Analog is read a single channel at a time,\non iterations 0 through 15."
                n137 = Unbundle(w275) -> ("Analog Module 1"=w276:bool[], "Analog Module 2"=w277:bool[])  [unwired: 3 out]
                n138 = Build Array (concatenate)(w276, w277) -> (w273:bool[])
                n139 = Index Array(array=w273, index=w272) -> (element=w274:bool)
                n140 = case shown="True" w274 {
                  tunnel: w272 -> [_ w289]
                  tunnel: [w278 w279] -> w271
                  tunnel: w269 -> [w278 _]
                  frame False {
                  }
                  frame True {
                    n141 = Quotient & Remainder(x=w289, y=8) -> (x-y*floor(x/y)=w286:i32, floor(x/y)=w290:i32)
                    n142 = Bundle("DevStatus"=errorcluster {"status"=FALSE, "code"=0, "source"=""}, w290) -> (w292:cluster{"DevStatus":errorcluster, i32})  [unwired: 1 out]
                    n143 = call <vilib>:"NT Read Numeric Array.vi"("Name"="analog") -> ("error out"=w281:errorcluster, "Numeric Array"=w287:dbl[])  [unwired: 9 in]
                    n144 = call <vilib>:"WPI_AnalogModuleGetAverageVoltage.vi"("Channel"=w286, "AnalogModuleDevStatus"=w292) -> ("error out"=w280:errorcluster, "Average Voltage"=w285:dbl)  [unwired: 1 in, 7 out]
                    n145 = Replace Array Subset(array=w287, new element=w285, index=w286) -> (w283:dbl[])
                    n146 = Merge Errors(w281, w280) -> (w282:errorcluster)
                    n147 = call <vilib>:"NT Write Numeric Array.vi"("error in"=w282, "Numeric Array"=w283, "Name"="analog") -> ("error out"=w279:errorcluster)  [unwired: 8 in]
                  }
                }
                n148 = Merge Errors(w271, w269) -> (w270:errorcluster)
              }
              frame Disabled {
                n149 = in-place {
                  n150 = in-place-cluster #7(w295) -> ()  [unwired: 1 out]
                  n151 = call "dash safety data FG.vi"("Menu"=fg_typedef."Get") -> ("Arm Safety Data Out"=w300:T9)  [unwired: 3 in, 1 out]
                  n152 = in-place-cluster #7("Arm Safety Data"=w300) -> (w294:T8)
                }
                n153 = Flatten To String(anything=w294) -> (data string=w298:string, error out=w296:errorcluster)  [unwired: 1 in, 3 out]
                n154 = call <vilib>:"NT Write String.vi"("error in"=w296, "String"=w298, "Name"="dashdata") -> ()  [unwired: 8 in, 1 out]
              }
            }
          }
          frame 25 {
            w318 = enum16{"set", "get"}."get" ("menu (get)")
            # "update subsystem states"
            n155 = call "states FG.vi"("menu (get)"=w318, "Loop ID"=0) -> ("subState out"=w315:T4)  [unwired: 6 in, 3 out]
            n156 = call "states FG.vi"("menu (get)"=w318, "Loop ID"=1) -> ("subState out"=w316:T4)  [unwired: 6 in, 3 out]
            n157 = call "states FG.vi"("menu (get)"=w318, "Loop ID"=2) -> ("subState out"=w317:T4)  [unwired: 6 in, 3 out]
            n158 = call "states FG.vi"("menu (get)"=w318, "Loop ID"=3) -> ("subState out"=w314:T4)  [unwired: 6 in, 3 out]
            n159 = call "states FG.vi"("menu (get)"=w318, "Loop ID"=4) -> ("subState out"=w313:T4)  [unwired: 6 in, 3 out]
            n160 = To Double Precision Float(number=w315) -> (double precision float=w311:dbl)
            n161 = To Double Precision Float(number=w316) -> (double precision float=w310:dbl)
            n162 = To Double Precision Float(number=w317) -> (double precision float=w309:dbl)
            n163 = To Double Precision Float(number=w314) -> (double precision float=w308:dbl)
            n164 = To Double Precision Float(number=w313) -> (double precision float=w307:dbl)
            n165 = Build Array(w311, w310, w309, w308, w307) -> (w306:dbl[])
            n166 = call <vilib>:"NT Write Numeric Array.vi"("Numeric Array"=w306, "Name"="subsystem_states") -> ("error out"=w305:errorcluster)  [unwired: 9 in]
            n167 = disable-structure shown="Enabled" {
              disable-tunnel: w305 -> [w326 _]
              disable-tunnel: [w325 w327] -> w304
              disable-tunnel: w303 -> [w324 w327]
              frame Disabled {
                n168 = Merge Errors(w326, w324) -> (w325:errorcluster)
              }
              frame Enabled {
              }
            }
          }
          frame 20, 30 {
            # "Digital I/O is pretty fast,\nso the values are read a module\nat a time, one module on call 20,\nanother on call 30."
            n169 = Equal?(x=30, y=w339) -> (x = y?=w336:bool)
            n170 = Boolean To (0,1)(Boolean=w336) -> (0, 1=w337:i16)
            n171 = Unbundle(w338) -> ("Digital Module 1"=w341:bool, "Digital Module 2"=w340:bool)  [unwired: 3 out]
            n172 = To Long Integer(number=w337) -> (32bit integer=w334:i32)
            n173 = Select(t=FPGA_TypedefDigitalModule."Digital Module 2" ("Module (Module 1)"), s=w336, f=FPGA_TypedefDigitalModule."Digital Module 1" ("Module (Module 1)")) -> (s? t:f=w333:T7)
            n174 = Build Array(w341, w340) -> (w342:bool[])
            n175 = Index Array(array=w342, index=w334) -> (element=w343:bool)
            n176 = case shown="True" w343 {
              tunnel: w333 -> [_ w359]
              tunnel: w334 -> [_ w358]
              tunnel: [errorcluster {"status"=FALSE, "code"=0, "source"=""} ("error out") w353] -> w331
              tunnel: w330 -> [_ _]
              frame False {
              }
              frame True {
                n177 = call <vilib>:"FPGA_DIOOpen.vi"("Module (Module 1)"=w359) -> ("DIODeviceRef"=w376:T20)  [unwired: 1 in, 9 out]
                n178 = for {
                  N: 10 -> [_]
                  tunnel: w376 -> [w386]
                  tunnel: [w384] -> w377 mode=indexing
                  i -> [w385]
                  n179 = To Unsigned Byte Integer(number=w385) -> (unsigned 8bit integer=w383:u8)
                  n180 = call <vilib>:"FPGA_DIOReadPWMValue.vi"("PWMChannel"=w383, "DIODeviceRef In"=w386) -> ("PWMValue"=w384:u8)  [unwired: 1 in, 8 out]
                }
                n181 = call <vilib>:"FPGA_DIOReadSlowValueRelayFwd.vi"("DIODeviceRef In"=w376) -> ("Relay Forward"=w369:u8)  [unwired: 1 in, 9 out]
                n182 = call <vilib>:"FPGA_DIOReadSlowValueRelayRev.vi"("DIODeviceRef In"=w376) -> ("Relay Reverse"=w370:u8)  [unwired: 1 in, 9 out]
                n183 = call <vilib>:"FPGA_DIOReadDI.vi"("DIODeviceRef In"=w376) -> ("DI"=w374:u16)  [unwired: 1 in, 9 out]
                n184 = call <vilib>:"FPGA_DIOReadDO.vi"("DIODeviceRef In"=w376) -> ("DO"=w373:u16)  [unwired: 1 in, 9 out]
                n185 = call <vilib>:"FPGA_DIOReadOutputEnable.vi"("DIODeviceRef In"=w376) -> ("OutputEnable"=w364:u16)  [unwired: 1 in, 9 out]
                n186 = And(x=w373, y=w364) -> (x .and. y?=w372:u16)
                n187 = Compound Arithmetic op=AND(w374, invert w364) -> (w371:u16)
                n188 = Number To Boolean Array(number=w364) -> (Boolean array=w366:bool[])
                n189 = Or(x=w371, y=w372) -> (x .or. y?=w362:u16)
                n190 = Reverse 1D Array(array=w366) -> (reversed array=w365:bool[])
                n191 = Number To Boolean Array(number=w362) -> (Boolean array=w367:bool[])
                n192 = Boolean Array To Number(Boolean array=w365) -> (number=w363:u32)
                n193 = Reverse 1D Array(array=w367) -> (reversed array=w368:bool[])
                n194 = Array To Cluster(array=w377) -> (cluster=w375:T21)
                n195 = Boolean Array To Number(Boolean array=w368) -> (number=w361:u32)
                n196 = To Unsigned Word Integer(number=w361) -> (unsigned 16bit integer=w350:u16)
                n197 = To Unsigned Word Integer(number=w363) -> (unsigned 16bit integer=w351:u16)
                n198 = Bundle(cluster=T2 {"Relay Fwd"=0, "Relay Rev"=0, "GPIO"=0, "GPIO_OE"=0, "PWM"={"PWM[0]"=0, "PWM[1]"=0, "PWM[2]"=0, "PWM[3]"=0, "PWM[4]"=0, "PWM[5]"=0, "PWM[6]"=0, "PWM[7]"=0, "PWM[8]"=0, "PWM[9]"=0}} ("DigitalModule"), "Relay Fwd"=w369, "Relay Rev"=w370, "GPIO"=w350, "GPIO_OE"=w351, "PWM"=w375) -> (w360:T2)
                n199 = disable-structure shown="Enabled" {
                  disable-tunnel: w360 -> [w381 w382]
                  disable-tunnel: w358 -> [w380 _]
                  disable-tunnel: [_ w382] -> w357
                  frame Disabled {
                    n200 = Replace Array Subset(array=T2[] [], new element=w381, index=w380) -> ()  [unwired: 1 out]
                  }
                  frame Enabled {
                  }
                }
                n201 = Flatten To String(anything=w357) -> (data string=w355:string, error out=w356:errorcluster)  [unwired: 1 in, 3 out]
                n202 = call <vilib>:"NT Write String.vi"("error in"=w356, "String"=w355, "Name"="dio") -> ("error out"=w353:errorcluster)  [unwired: 8 in]
              }
            }
            n203 = disable-structure shown="Enabled" {
              disable-tunnel: w331 -> [w347 _]
              disable-tunnel: w330 -> [w346 w348]
              disable-tunnel: [w345 w348] -> w329
              frame Disabled {
                n204 = Merge Errors(w347, w346) -> (w345:errorcluster)
              }
              frame Enabled {
              }
            }
          }
          frame 32 {
            # "update encoders"
            n205 = call <vilib>:"WPI_EncoderRefNum Registry Get.vi"("refnum name"="pickup arm") -> ("error out"=w400:errorcluster, "EncoderDevRef"=w399:T27)  [unwired: 9 in]
            n206 = call <vilib>:"WPI_EncoderRefNum Registry Get.vi"("refnum name"="right") -> ("error out"=w405:errorcluster, "EncoderDevRef"=w404:T27)  [unwired: 9 in]
            n207 = call <vilib>:"WPI_EncoderRefNum Registry Get.vi"("refnum name"="left") -> ("error out"=w402:errorcluster, "EncoderDevRef"=w403:T27)  [unwired: 9 in]
            n208 = call <vilib>:"WPI_EncoderGet.vi"("error in (no error)"=w405, "EncoderDevRef"=w404) -> ("Distance"=w397:dbl, "Rate"=w396:dbl)  [unwired: 4 in, 4 out]
            n209 = call <vilib>:"WPI_EncoderGet.vi"("error in (no error)"=w402, "EncoderDevRef"=w403) -> ("Distance"=w395:dbl, "Rate"=w394:dbl)  [unwired: 4 in, 4 out]
            n210 = call <vilib>:"WPI_EncoderGet.vi"("error in (no error)"=w400, "EncoderDevRef"=w399) -> ("Distance"=w393:dbl, "Rate"=w392:dbl)  [unwired: 4 in, 4 out]
            n211 = Build Array(w397, w396, w395, w394, w393, w392) -> (w391:dbl[])
            n212 = call <vilib>:"NT Write Numeric Array.vi"("Numeric Array"=w391, "Name"="encoders") -> ("error out"=w390:errorcluster)  [unwired: 9 in]
            n213 = disable-structure shown="Enabled" {
              disable-tunnel: w390 -> [w410 _]
              disable-tunnel: [w409 w411] -> w389
              disable-tunnel: w388 -> [w408 w411]
              frame Disabled {
                n214 = Merge Errors(w410, w408) -> (w409:errorcluster)
              }
              frame Enabled {
              }
            }
          }
          frame 37 {
            # "update motor array"
            n215 = call <vilib>:"WPI_MotorControlRefNum Registry Get.vi"("refnum name"="belts") -> ("error out"=w419:errorcluster, "MotorControlDevRef"=w421:T31)  [unwired: 9 in]
            n216 = call <vilib>:"WPI_MotorControlGetOutput.vi"("error in (no error)"=w419, "MotorControlDevRef"=w421) -> ("error out"=w414:errorcluster, "Output"=w418:dbl)  [unwired: 7 in, 1 out]
            n217 = call <vilib>:"NT Write Number.vi"("error in"=w414, "Numeric"=w418, "Name"="belts") -> ("error out"=w413:errorcluster)  [unwired: 8 in]
            n218 = disable-structure shown="Enabled" {
              disable-tunnel: [w424 w425] -> w416
              disable-tunnel: w415 -> [w423 w425]
              disable-tunnel: w413 -> [w422 _]
              frame Disabled {
                n219 = Merge Errors(w423, w422) -> (w424:errorcluster)
              }
              frame Enabled {
              }
            }
          }
          frame 40 {
            # "The solenoids are pretty fast, so all are read on call 40."
            n220 = Unbundle(w447) -> ("Solenoid Module"=w448:bool)  [unwired: 4 out]
            n221 = call <vilib>:"NT Read Number.vi"("Name"="solenoids") -> ("error out"=w437:errorcluster, "Numeric"=w444:dbl)  [unwired: 9 in]
            n222 = To Unsigned Byte Integer(number=w444) -> (unsigned 8bit integer=w442:u8)
            n223 = call <vilib>:"WPI_CompressorRefNum Registry Get.vi"("refnum name"="compressor") -> ("error out"=w434:errorcluster, "CompressorDevRef"=w433:T39)  [unwired: 9 in]
            n224 = case shown="True" w448 {
              tunnel: [w455 w459] -> w446
              tunnel: w442 -> [w455 _]
              tunnel: [w454 w457] -> w438
              tunnel: w437 -> [w454 w456]
              frame False {
              }
              frame True {
                n225 = call <vilib>:"FPGA_SolenoidOpen.vi"("error in (no error)"=w456) -> ("error out"=w458:errorcluster, "SolenoidDevRef"=w460:T22)  [unwired: 1 in, 8 out]
                n226 = call <vilib>:"FPGA_SolenoidReadD07_0.vi"("error in (no error)"=w458, "SolenoidDevRef"=w460) -> ("error out"=w457:errorcluster, "DO7:0"=w459:u8)  [unwired: 8 out]
              }
            }
            n227 = call "compressor_getenablstate.vi"("error in (no error)"=w434, "CompressorDevRef"=w433) -> ("error out"=w426:errorcluster, "Compressor Running"=w430:bool, "Enabled"=w431:bool)  [unwired: 6 in, 1 out]
            n228 = Build Array(w431, w430) -> (w429:bool[])
            n229 = call <vilib>:"NT Write Boolean Array.vi"("error in"=w426, "Boolean Array"=w429, "Name"="compressor") -> ("error out"=w427:errorcluster)  [unwired: 8 in]
            n230 = To Double Precision Float(number=w446) -> (double precision float=w441:dbl)
            n231 = call <vilib>:"NT Write Number.vi"("error in"=w438, "Numeric"=w441, "Name"="solenoids") -> ("error out"=w439:errorcluster)  [unwired: 8 in]
            n232 = disable-structure shown="Disabled" {
              disable-tunnel: [w452 w453] -> w440
              disable-tunnel: w439 -> [w451 _]
              disable-tunnel: w436 -> [w450 w453]
              disable-tunnel: w427 -> [w449 _]
              frame Disabled {
                n233 = Merge Errors(w451, w450, w449) -> (w452:errorcluster)
              }
              frame Enabled {
              }
            }
          }
          frame 45 {
            w479 = fg_typedef."Get" ("Menu")
            n234 = call "dash safety data FG.vi"("Menu"=w479) -> ("Drive Safety Data Out"=w461:T10, "Arm Safety Data Out"=w462:T9)  [unwired: 3 in]
            n235 = call <vilib>:"RT Get CPU Loads.vi"() -> ("error out"=w469:errorcluster, "CPU loads"=w484:T37[])  [unwired: 10 in]
            n236 = call "performance fg.vi"("Menu"=w479) -> ("Output"=w483:T38)  [unwired: 1 in]
            n237 = call "vision data fg.vi"("Menu"=w479) -> ("Output"=w482:T15)  [unwired: 1 in]
            n238 = call "vision_fg.vi"("Menu"=w479) -> ("Enabled?"=w477:bool)  [unwired: 2 in, 1 out]
            n239 = Unbundle(w482) -> ("Hot Goal Present?"=w481:bool, "distance"=w480:dbl)  [unwired: 5 out]
            n240 = Index Array(array=w484) -> (element=w485:T37)  [unwired: 1 in]
            n241 = call "match info fg.vi"("Menu (Set)"=enum16{"Get", "Set"}."Get") -> ("TeleOp Elapsed Seconds"=w463:dbl)  [unwired: 26 in]
            n242 = Unbundle By Name(w485) -> ("Total (%)"=w473:dbl)
            n243 = Unbundle By Name(w483) -> ("Vision mSPI"=w474:u32, "Main mSPI"=w475:u32)
            n244 = Bundle("Hot Goal Present?"=w481, "distance"=w480) -> (w476:T26)  [unwired: 1 in]
            n245 = Bundle By Name(cluster=T8 {"Total (%)"=0.0, "Vision mSPI"=0, "Main mSPI"=0, "Vision"={"Hot Goal Present?"=FALSE, "distance"=0.0}, "Enabled?"=FALSE, "Arm Safety Data"={"At Distance Limit"=FALSE, "No Rate Read"=FALSE, "Encoder Failure"=FALSE, "Encoder Directional Issue"=FALSE}, "Drive Safety Data"={"Left - Encoder Failure"=FALSE, "Left - No Rate Read"=FALSE, "Right - Encoder Failure"=FALSE, "Right - No Rate Read"=FALSE}, "TeleOp Elapsed Seconds"=0.0}, "TeleOp Elapsed Seconds"=w463, "Arm Safety Data"=w462, "Drive Safety Data"=w461, "Total (%)"=w473, "Vision mSPI"=w474, "Main mSPI"=w475, "Vision"=w476, "Enabled?"=w477) -> (w465:T8)
            n246 = Flatten To String(anything=w465, error in (no error)=w469) -> (data string=w472:string, error out=w470:errorcluster)  [unwired: 3 out]
            n247 = call <vilib>:"NT Write String.vi"("error in"=w470, "String"=w472, "Name"="dashdata") -> ("error out"=w468:errorcluster)  [unwired: 8 in]
            n248 = disable-structure shown="Enabled" {
              disable-tunnel: w468 -> [w488 _]
              disable-tunnel: [w487 w489] -> w467
              disable-tunnel: w466 -> [w486 w489]
              frame Disabled {
                n249 = Merge Errors(w488, w486) -> (w487:errorcluster)
              }
              frame Enabled {
              }
            }
          }
          frame 47 {
            n250 = call "timeout error fg.vi"() -> ("# of Timeouts"=w503:u32, "Time Out Error This Match"=w502:bool)  [unwired: 2 in]
            n251 = call "safe shoot error.vi"("Menu"=fg_typedef."Get") -> ("Can Shoot Safely?"=w499:bool)  [unwired: 1 in]
            n252 = Bundle By Name(cluster=T6 {"# of Timeouts"=0, "Time Out Error This Match"=FALSE}, "Time Out Error This Match"=w502, "# of Timeouts"=w503) -> (w500:T6)
            n253 = Bundle By Name(cluster=T11 {"Timeout Data"={"# of Timeouts"=0, "Time Out Error This Match"=FALSE}, "Can Shoot Safely?"=FALSE}, "Timeout Data"=w500, "Can Shoot Safely?"=w499) -> (w498:T11)
            n254 = Flatten To String(anything=w498) -> (data string=w494:string, error out=w496:errorcluster)  [unwired: 1 in, 3 out]
            n255 = call <vilib>:"NT Write String.vi"("error in"=w496, "String"=w494, "Name"="errors") -> ("error out"=w492:errorcluster)  [unwired: 8 in]
            n256 = disable-structure shown="Enabled" {
              disable-tunnel: [w507 w508] -> w493
              disable-tunnel: w492 -> [w506 _]
              disable-tunnel: w491 -> [w505 w508]
              frame Disabled {
                n257 = Merge Errors(w506, w505) -> (w507:errorcluster)
              }
              frame Enabled {
              }
            }
          }
        }
      }
      "Errors" <- w241
      n258 = First Call?() -> (First Call?: T/F=w240:bool)
      n259 = case shown="True" w240 {
        frame False {
        }
        frame True {
          n260 = call <vilib>:"NT Write String.vi"("String"="2014_05_07_v1", "Name"="code_rev") -> ()  [unwired: 9 in, 1 out]
        }
      }
    }
  }
